vi "play_nPoint_id_slew.vi"() -> ()   [LabVIEW 2017]
uses:
  <vilib>/userdefined/High Color/nirio_resource_hc.ctl
  <vilib>/FPGAPlugInAG/cRIO-9082/niLvFpga_Open_cRIO-9082.vi
  <vilib>/rvi/interface/common/dynamic/niFpgaDynamicAddResources.vi
  <vilib>/FPGAPlugInAG/Dynamic/niLvFpga_Reset_Dynamic.vi
  <vilib>/rvi/interface/common/niFpgaWaitOnOcc.vi
  <vilib>/Utility/error.llb/Error Cluster From Error Code.vi
  <vilib>/rvi/errors/niLvFpgaAdjustHostInterfaceError.vi
  <vilib>/FPGAPlugInAG/Dynamic/niLvFpga_Run_Dynamic.vi
  <vilib>/Utility/file.llb/Write Delimited Spreadsheet (DBL).vi
  <vilib>/FPGAPlugInAG/Dynamic/niLvFpga_Close_Dynamic.vi
  <vilib>/rvi/interface/nirviOpenFPGA/nirviOpenFPGA.xnode
  FPGA Bitfiles/XYpeizocontrol_FPGATargetSPARTA_nPointidslew_8MQm-sFNxL4.lvbitx
  <vilib>/rvi/interface/nirviMethod/nirviMethod.xnode
  <vilib>/rvi/interface/nirviReadWriteControl/nirviReadWriteControl.xnode
  <vilib>/rvi/interface/nirviCloseFPGA/nirviCloseFPGA.xnode
  <vilib>/FPGAPlugInAG/Dynamic/niLvFpga_ConfigureFifo_Dynamic.vi
  <vilib>/rvi/errors/niLvFpgaMergeErrorWithErrorCode.vi
  <vilib>/rvi/interface/Simulation/niFpgaSimulationCallBeginRW.vi
  <vilib>/FPGAPlugInAG/Dynamic/niLvFpga_ReadFifo_Dynamic.vi
  NiFpgaLv.dll
panel:
  out "AI0":dbl[](array[numeric])
  out "AI1":dbl[](array[numeric])
  out "AI1":T1(graph)
  out "size(s) 2":i32[](array[numeric])
  in  "file path (dialog if empty)":path
  out "AI0":T1(graph)
  out "Waveform Chart":T1(graph)
  out "Loop Done":bool
  in  "Abort":bool
  in  "TsTicks":u32=1600
  in  "yref_k":sgl min=-5 max=5 step=0.1
  out "y iter":i32
  out "size(s)":i32
  in  "ymax":dbl=4.0 format="%#_13g"
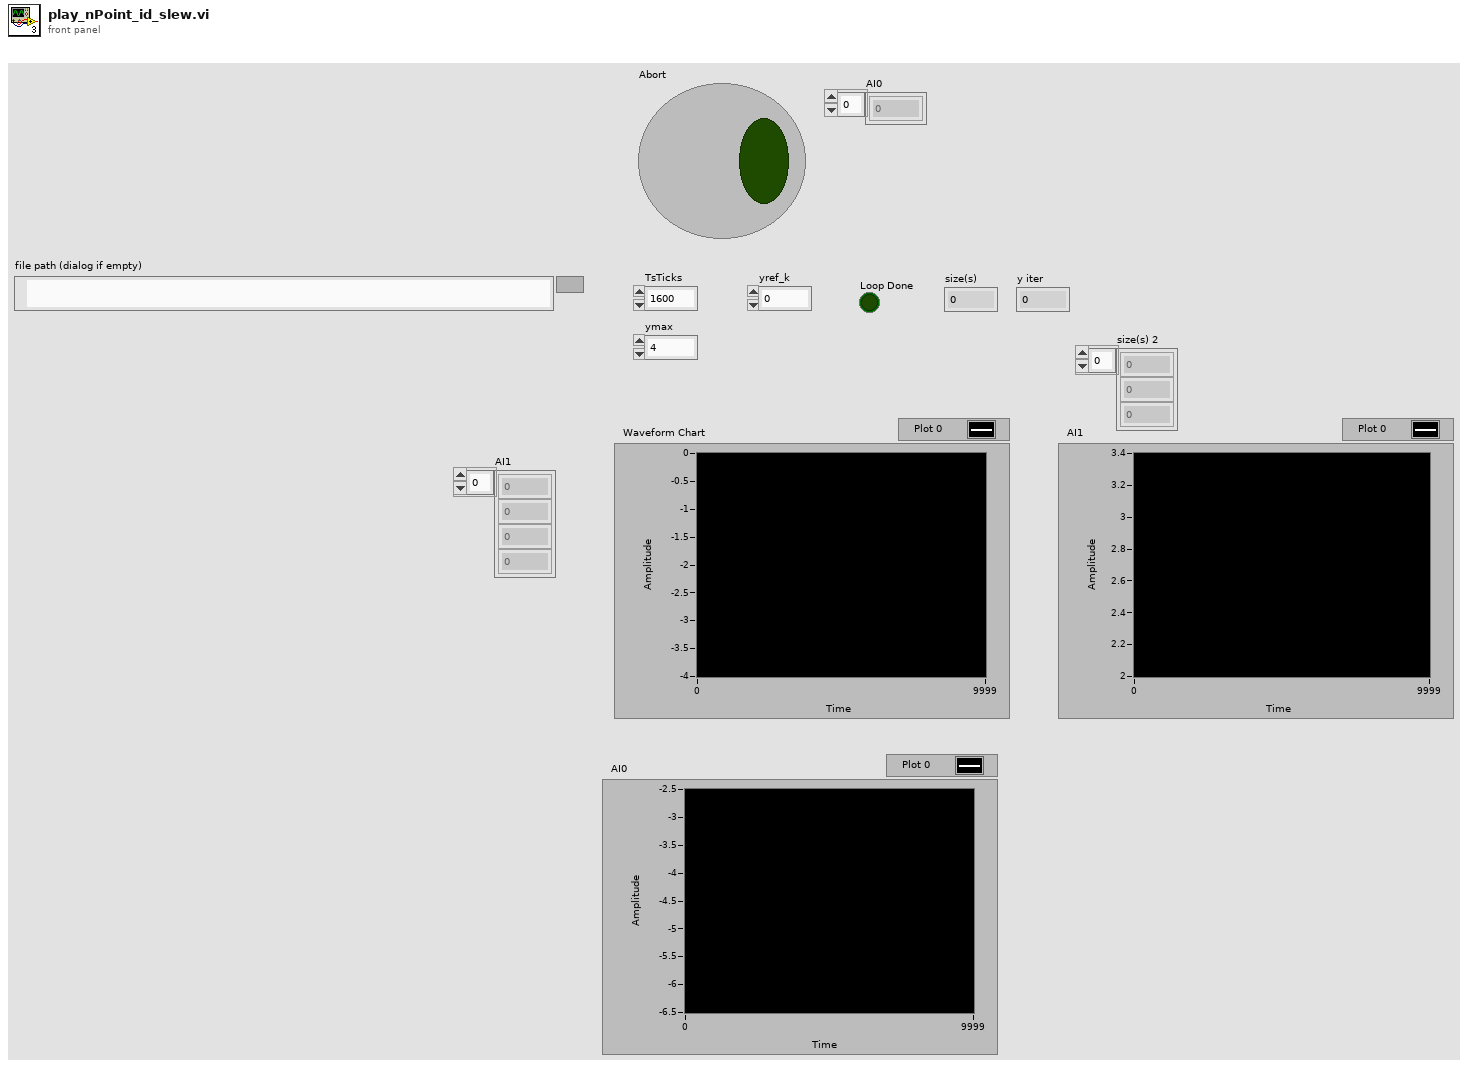
[diagram p1: front panel]
types:
  T1 = cluster{"2D Data Out[0]":dbl, "2D Data Out[1]":dbl, "2D Data Out[2]":dbl, "2D Data Out[3]":dbl, "2D Data Out[4]":dbl, "2D Data Out[5]":dbl, "2D Data Out[6]":dbl, "2D Data Out[7]":dbl, "2D Data Out[8]":dbl}
  T2 = typedef "nirio_resource_hc.ctl" = tag
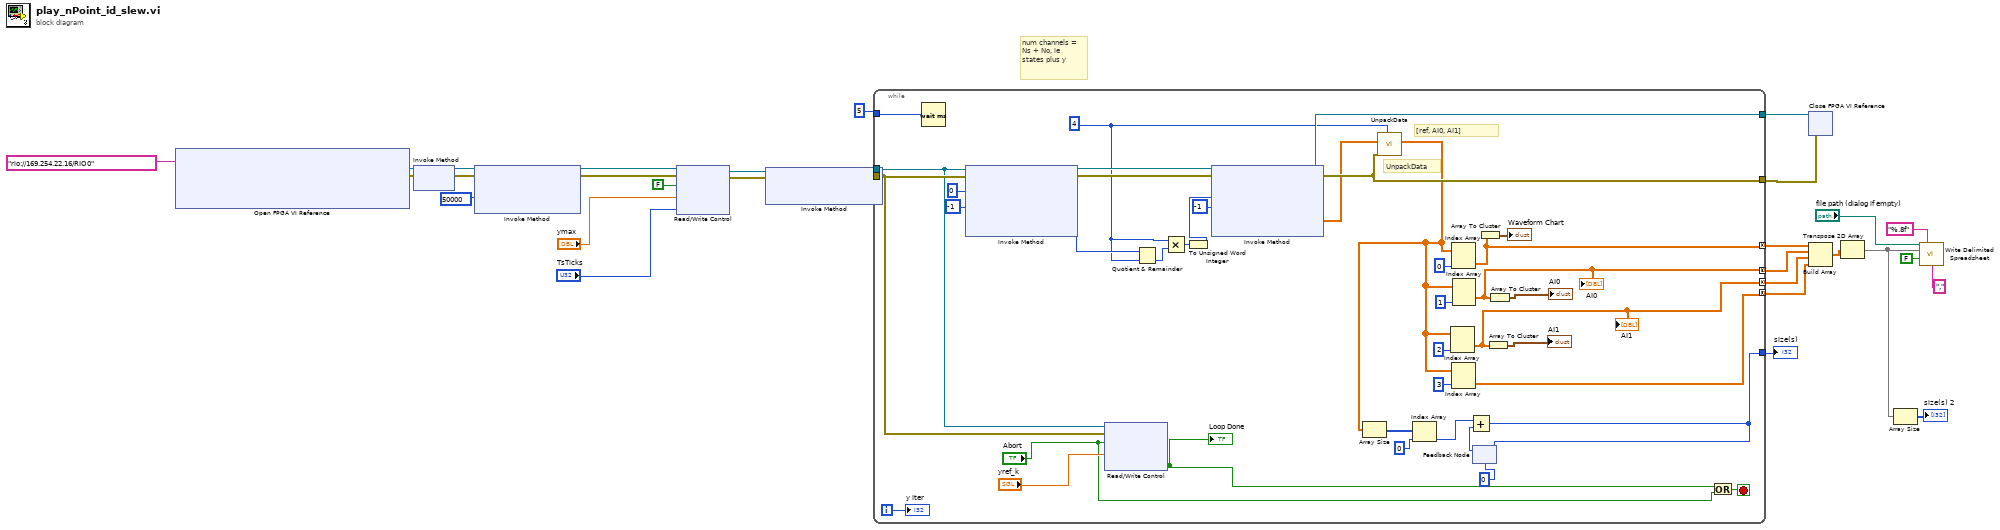
[diagram p0: block diagram]
diagram:
  # "num channels = Ns + No, ie states plus y"
  n1 = xnode "Open FPGA VI Reference"("resource name"=T2 "rio://169.254.22.16/RIO0") -> ("FPGA VI Reference Out"=w26:refnum<k20>, "error out"=w25:errorcluster)  [unwired: 1 in]
  n2 = xnode "Invoke Method"("FPGA VI Reference In"=w26, "error in"=w25) -> ("FPGA VI Reference Out"=w18:refnum<k20>, "error out"=w17:errorcluster)
  n3 = xnode "Invoke Method"("FPGA VI Reference In"=w18, "error in"=w17, "Requested Depth"=50000) -> ("FPGA VI Reference Out"=w13:refnum<k20>, "error out"=w14:errorcluster)  [unwired: 1 out]
  n4 = xnode "Read/Write Control"("FPGA VI Reference In"=w13, "error in"=w14, "Abort"=FALSE, "ymax"="ymax", "TsTicks"="TsTicks") -> ("FPGA VI Reference Out"=w21:refnum<k20>, "error out"=w20:errorcluster)
  n5 = xnode "Invoke Method"("FPGA VI Reference In"=w21, "error in"=w20) -> ("FPGA VI Reference Out"=w23:refnum<k20>, "error out"=w22:errorcluster)  [unwired: 1 in]
  n6 = while {
    tunnel: 5 -> [w69]
    tunnel: w23 -> [w46]
    tunnel: w22 -> [w47]
    tunnel: [w61] -> w15
    tunnel: [w60] -> w28
    tunnel: [w50] -> w27
    tunnel: [w38] -> w11 mode=concatenating
    tunnel: [w37] -> w10 mode=concatenating
    tunnel: [w34] -> w2 mode=concatenating
    tunnel: [w31] -> w1 mode=concatenating
    i -> [w51]
    stop <- w49 stop-if-true
    w48 = u32 4 ("y")
    # "[ref, AI0, AI1]"
    # "UnpackData"
    n7 = Wait (ms)(milliseconds to wait=w69) -> ()  [unwired: 1 out]
    n8 = xnode "Invoke Method"("FPGA VI Reference In"=w46, "error in"=w47, "Number of Elements"=0 ("Timeout (ms)"), "Timeout (ms)"=-1) -> ("FPGA VI Reference Out"=w65:refnum<k20>, "error out"=w66:errorcluster, "Elements Remaining"=w57:u32)  [unwired: 1 out]
    n9 = xnode "Read/Write Control"("FPGA VI Reference In"=w46, "error in"=w47, "Abort"="Abort", "yref_k"="yref_k") -> ("Loop Done"=w43:bool)  [unwired: 2 out]
    "Loop Done" <- w43
    n10 = Quotient & Remainder(x=w57, y=w48) -> (floor(x/y)=w58:u32)  [unwired: 1 out]
    n11 = Multiply(x=w48, y=w58) -> (x*y=w63:u32)
    n12 = To Unsigned Word Integer(number=w63) -> (unsigned 16bit integer=w59:u16)
    n13 = xnode "Invoke Method"("FPGA VI Reference In"=w65, "error in"=w66, "Number of Elements"=w59, "Timeout (ms)"=-1) -> ("FPGA VI Reference Out"=w60:refnum<k20>, "error out"=w61:errorcluster, "Data"=w56:sgl[])  [unwired: 1 out]
    n14 = call "UnpackData.vi"("NumChannels"=w48, "error In"=w61, "1D Data In"=w56) -> ("2D Data Out"=w33:dbl[][])  [unwired: 7 in, 1 out]
    n15 = Array Size(array=w33) -> (size(s)=w55:i32[])
    n16 = Index Array(array=w55, index=0) -> (element=w53:i32)
    n17 = Index Array(array=w33, index (col)=2 ("disabled index (col)")) -> (element=w34:dbl[])  [unwired: 1 in]
    "AI1" <- w34
    n18 = Index Array(array=w33, index (col)=0 ("disabled index (col)")) -> (element=w38:dbl[])  [unwired: 1 in]
    n19 = Index Array(array=w33, index (col)=3 ("disabled index (col)")) -> (element=w31:dbl[])  [unwired: 1 in]
    n20 = Index Array(array=w33, index (col)=1 ("disabled index (col)")) -> (element=w37:dbl[])  [unwired: 1 in]
    "AI0" <- w37
    n21 = feedback #1(0) -> (w54:i32)
    n22 = Add(x=w53, y=w54) -> (x+y=w50:i32)
    n23 = feedback-in #1(w50) -> ()
    n24 = Array To Cluster(array=w38) -> (cluster=→"Waveform Chart":T1)
    n25 = Array To Cluster(array=w34) -> (cluster=→"AI1":T1)
    n26 = Array To Cluster(array=w37) -> (cluster=→"AI0":T1)
    n27 = Or(x=w43, y="Abort") -> (x .or. y?=w49:bool)
    "y iter" <- w51
  }
  "size(s)" <- w27
  n28 = xnode "Close FPGA VI Reference"("FPGA VI Reference In"=w28, "error in"=w15) -> ()  [unwired: 1 out]
  n29 = Build Array(w11, w10, w2, w1) -> (w4:dbl[][])
  n30 = Transpose 2D Array(2D array=w4) -> (transposed array=w3:dbl[][])
  n31 = Array Size(array=w3) -> (size(s)=→"size(s) 2":i32[])
  n32 = call-poly <vilib>:"Write Delimited Spreadsheet.vi"("file path (dialog if empty)"="file path (dialog if empty)", "format (%.3f)"="%.8f", "2D data"=w3, "append to file? (new file:F)"=FALSE, "delimiter (\\t)"="," ("delimiter (\\t)")) -> ()  [unwired: 9 in, 2 out]
